vi "Read Data.vi"(8 "error in (no error)":errorcluster, 11 "handle in":u32) -> (0 "error out":errorcluster, 2 "Data Buffer":u16[](array[numeric]), 3 "handle out":u32)   [LabVIEW 2016, in "Photon Counter.lvlib" / "C8855-01.lvlib"]
doc: "Reads out the counter data from this unit in the transfer mode specified by Setup.\n\n\n\n\nBOOL C8855API __stdcall C8855ReadData( HANDLE hC8855,\n DWORD *DataBuffer,\n BYTE *ResultReturned );"
uses:
  C8855-01.lvlib
  C8855-01api.dll
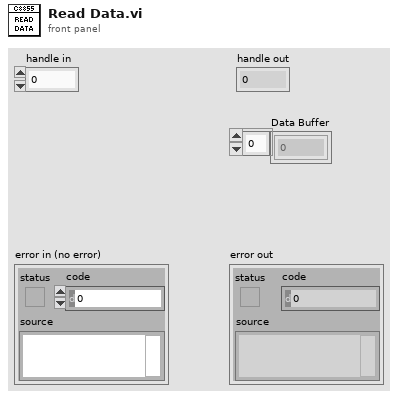
[diagram p1: front panel]
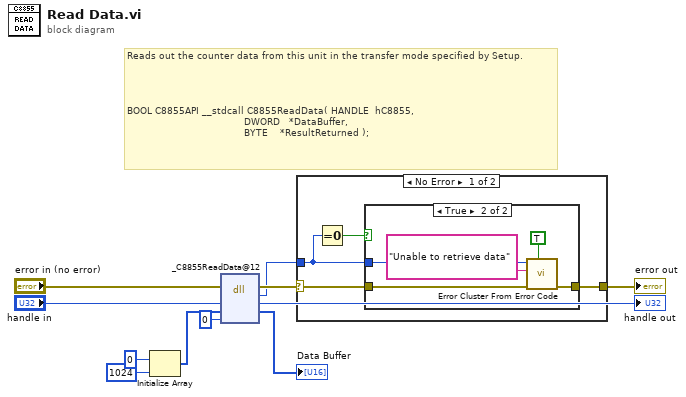
[diagram p0: block diagram]
diagram:
  # "Reads out the counter data from this unit in the transfer mode specified by Setup.\n\n\n\n\nBOOL C8855API __stdcall C8855ReadData( HANDLE  hC8855,\n                                       DWORD   *DataBuffer,\n                                       BYTE    *ResultReturned );"
  n1 = Initialize Array(u16 0 ("element"), 1024 ("dimension size")) -> (w1:u16[])
  n2 = dll-call lib="Z:/VM Shared Folder/Trace Grabber/Drivers/C8855-01/C8855-01api.*" fn="_C8855ReadData@12"(error in="error in (no error)", "Handle"="handle in", "Data Buffer"=w1, "Result Returned"=u8 0) -> (error out=w6:errorcluster, "return type"=w5:i32, "Handle"=→"handle out":u32, "Data Buffer"=→"Data Buffer":u16[])  [unwired: 3 in, 1 out]
  n3 = case shown="No Error" w6 {
    selector: w6 -> [w14 w22]
    tunnel: w5 -> [w12 _]
    tunnel: [w13 w22] -> w4
    frame No Error {
      n4 = Equal To 0?(x=w12) -> (x = 0?=w15:bool)
      n5 = case shown="True" w15 {
        tunnel: w14 -> [w16 w20]
        tunnel: [w16 w19] -> w13
        tunnel: w12 -> [_ w18]
        frame False {
        }
        frame True {
          n6 = call <vilib>:"Error Cluster From Error Code.vi"("show call chain? (False)"=TRUE, "error in (no error)"=w20, "error message (\"\")"="Unable to retrieve data" ("error message (\"\")"), "error code (0)"=w18) -> ("error out"=w19:errorcluster)  [unwired: 5 in]
        }
      }
    }
    frame Error {
    }
  }
  "error out" <- w4
